vi "Create Prism Color Map.vi"(1 "Size":i32) -> (0 "Colors":u32[](array[colorbox]))   [LabVIEW 2020]
uses:
  LinSpace (x0-dx-npts).vi
  481415bf-1445-4403-b7f3-31709fb4ea01.vi
  bd040a9e-2d90-4db6-8cbf-37cf07de0079.vi
  ba7a57c9-d8a4-48a8-917f-11fa72d785f8.vi
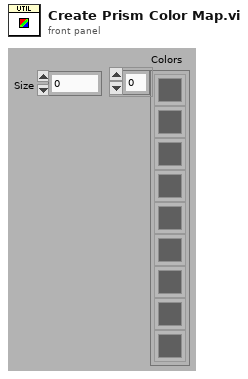
[diagram p1: front panel]
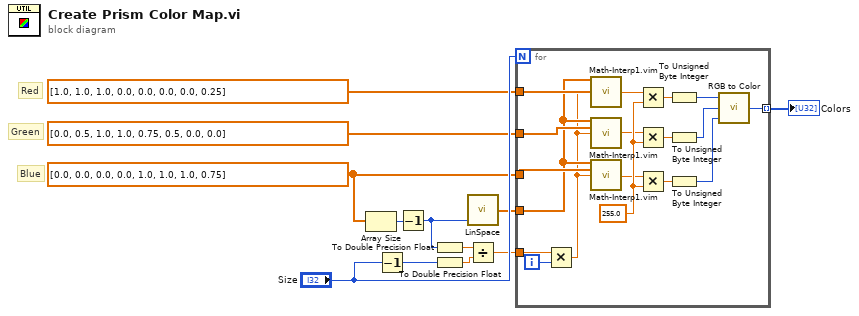
[diagram p0: block diagram]
diagram:
  w6 = dbl[] [0.0, 0.0, 0.0, 0.0, 1.0, 1.0, 1.0, 0.75]
  # "Blue"
  # "Green"
  # "Red"
  n1 = Array Size(array=w6) -> (size(s)=w11:i32)
  n2 = Decrement(x="Size") -> (x-1=w12:i32)
  n3 = Decrement(x=w11) -> (x-1=w1:i32)
  n4 = To Double Precision Float(number=w1) -> (double precision float=w3:dbl)
  n5 = To Double Precision Float(number=w12) -> (double precision float=w2:dbl)
  n6 = call-poly "LinSpace.vi"("npts"=w1) -> ("Array"=w5:dbl[])  [unwired: 3 in, 1 out]
  n7 = Divide(x=w3, y=w2) -> (x/y=w7:dbl)
  n8 = for {
    N: "Size" -> [_]
    tunnel: dbl[] [1.0, 1.0, 1.0, 0.0, 0.0, 0.0, 0.0, 0.25] -> [w30]
    tunnel: dbl[] [0.0, 0.5, 1.0, 1.0, 0.75, 0.5, 0.0, 0.0] -> [w29]
    tunnel: w6 -> [w28]
    tunnel: w7 -> [w26]
    tunnel: w5 -> [w25]
    tunnel: [w17] -> w4 mode=indexing
    i -> [w27]
    w24 = 255.0
    n9 = Multiply(x=w26, y=w27) -> (x*y=w13:dbl)
    n10 = call "Math-Interp1.vim"("X"=w25, "Y"=w30, "U"=w13) -> ("V"=w14:dbl)  [unwired: 12 in]
    n11 = call "Math-Interp1.vim"("X"=w25, "Y"=w29, "U"=w13) -> ("V"=w15:dbl)  [unwired: 12 in]
    n12 = call "Math-Interp1.vim"("X"=w25, "Y"=w28, "U"=w13) -> ("V"=w16:dbl)  [unwired: 12 in]
    n13 = Multiply(x=w14, y=w24) -> (x*y=w23:dbl)
    n14 = Multiply(x=w15, y=w24) -> (x*y=w22:dbl)
    n15 = Multiply(x=w16, y=w24) -> (x*y=w21:dbl)
    n16 = To Unsigned Byte Integer(number=w23) -> (unsigned 8bit integer=w20:u8)
    n17 = To Unsigned Byte Integer(number=w22) -> (unsigned 8bit integer=w19:u8)
    n18 = To Unsigned Byte Integer(number=w21) -> (unsigned 8bit integer=w18:u8)
    n19 = call <vilib>:"RGB to Color.vi"("B"=w18, "G"=w19, "R"=w20) -> ("Color"=w17:u32)
  }
  "Colors" <- w4
